vi "Lockin.GetStaticDependencies.vi"(8 "error in (no error)":errorcluster, 11 "Lockin":refnum<class "Lockin.lvclass">) -> (0 "error out":errorcluster, 2 "Dependencies":T1, 3 "Lockin out":refnum<class "Lockin.lvclass">)   [LabVIEW 2016, in "Lockin.lvclass"]
doc: "---------------------------------------------------------------\nJKI State Machine Objects™\nhttp://jki.net/state-machine-objects/\nCopyright (C) 2005-2015, JKI <info@jki.net>\nALL RIGHTS RESERVEDJKI State Machine Objects (SMO) 1.0.0.5\nJKI - JKI\nCopyright (c) 2016, JKI"
uses:
  Lockin.lvclass
  C:/Program Files (x86)/National Instruments/LabVIEW 2016/vi.lib/JKI/JKI SMO/SMO/SMO.lvclass
  Typedefs/Dependencies--Cluster.ctl
  <vilib>/JKI/JKI SMO/SMO/SMO.lvclass
panel:
  # "For instructions on how to use the JKI State Machine Objects, examples and video tutorials, visit:\nhttp://jki.net/state-machine-objects/\n\nJKI State Machine Objects™\nhttp://jki.net/state-machine-objects/\nCopyright (C) 2005-2015, JKI <info@jki.net>\nALL RIGHTS RESERVED"
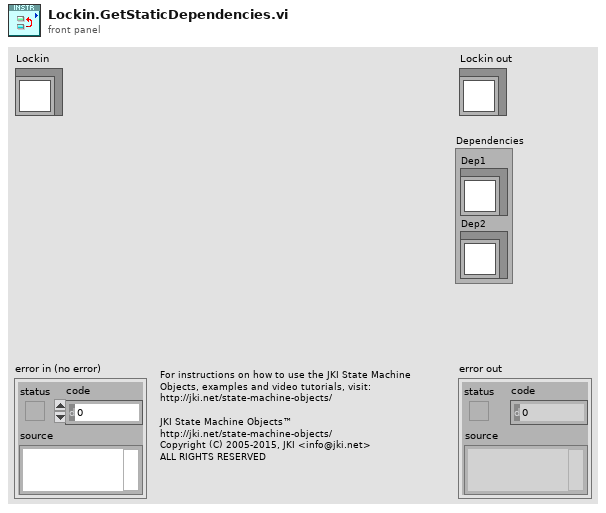
[diagram p1: front panel]
types:
  T1 = typedef "Lockin.lvclass/Dependencies--Cluster.ctl" = cluster{"Dep1":refnum<class "SMO.lvclass">, "Dep2":refnum<class "SMO.lvclass">}
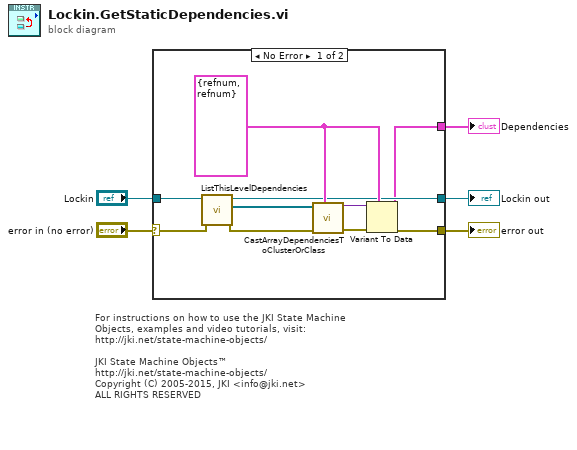
[diagram p0: block diagram]
diagram:
  # "For instructions on how to use the JKI State Machine Objects, examples and video tutorials, visit:\nhttp://jki.net/state-machine-objects/\n\nJKI State Machine Objects™\nhttp://jki.net/state-machine-objects/\nCopyright (C) 2005-2015, JKI <info@jki.net>\nALL RIGHTS RESERVED"
  n1 = case shown="No Error" "error in (no error)" {
    selector: "error in (no error)" -> [w6 w16]
    tunnel: "Lockin" -> [w15 w17]
    tunnel: [w8 w16] -> w4
    tunnel: [w9 w17] -> w3
    tunnel: [w7 _] -> w1
    frame No Error {
      w10 = T1 {"Dep1"=refnum, "Dep2"=refnum} ("Dependencies")
      n2 = call <vilib>:"ListThisLevelDependencies.vi"("error in (no error)"=w6, "SMO in"=w15) -> ("error out"=w13:errorcluster, "[My Dependencies]"=w14:refnum<class "SMO.lvclass">[], "SMO out"=w9:refnum<class "Lockin.lvclass">)  [unwired: 7 in]
      n3 = call <vilib>:"CastArrayDependenciesToClusterOrClass.vi"("Dependency Type (Class|Cluster)"=w10, "error in (no error)"=w13, "[Dependencies]"=w14) -> ("error out"=w12:errorcluster, "Dependencies output"=w11:variant)  [unwired: 7 in]
      n4 = Variant To Data(error in=w12, type=w10, Variant=w11) -> (data=w7:T1, error out=w8:errorcluster)
    }
    frame Error {
    }
  }
  "error out" <- w4
  "Lockin out" <- w3
  "Dependencies" <- w1
